vi "Gradient Ascent.vi"(0 "Function":enum16{"Reset", "Ascend"}(ring)=enum."Ascend", 1 "Set Inverse Matrix":T2=[[1.0, 0.0, 0.0], [0.0, 1.0, 0.0], [0.0, 0.0, 1.0]], 5 "Target Data":T1, 7 "Current Data":T1={"Match"={"Position"={"x"=0.0, "y"=0.0}, "Angle"=0.0, "Scale"=0.0, "Score"=0.0, "Bounding Box"=[]}, "Edge Analysis"={"Mean Value"=nan, "Standard Variation"=0.0, "Minimal Value"=0.0, "Maximal Value"=0.0, "Area (calibrated)"=0.0, "Area (pixels)"=0, "%"=0.0}}, 9 "Z":dbl=0.02, 11 "error in (no error)":errorcluster, 12 "Delta Z0":dbl=0.02, 14 "Alpha":dbl=0.01) -> (6 "Position Correction":dbl[](array[numeric]), 10 "Delta Z":dbl, 15 "error out":errorcluster)   [LabVIEW 2014]
uses:
  <vilib>/Analysis/Matrix/Datatypes/RealMatrix.ctl
  <vilib>/Analysis/baseanly.llb/A x Vector.vi
  <vilib>/Analysis/NI_AALBase.lvlib
  <vilib>/Analysis/NI_AALPro.lvlib
  <vilib>/Analysis/Matrix/NI_Matrix.lvlib
panel:
  out "Step Counter":i32
  out "Slope Fit":cluster{"Best Linear Fit":dbl[], sgl[]}[](graph)
  # "LICENSED MATERIALS – PROPERTY OF IBM\nCopyright IBM Corp. 2016, 2016\nALL RIGHTS RESERVED"
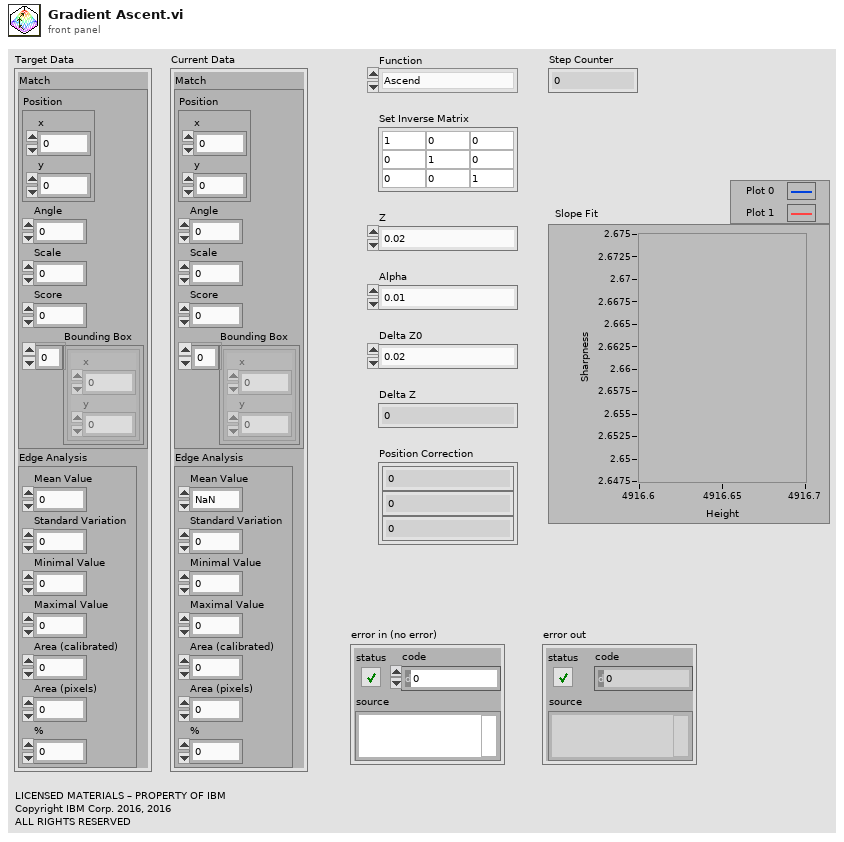
[diagram p1: front panel]
types:
  T1 = cluster{"Match":cluster{"Position":cluster{"x":sgl, "y":sgl}, "Angle":sgl, "Scale":sgl, "Score":sgl, "Bounding Box":cluster{"x":sgl, "y":sgl}[]}, "Edge Analysis":cluster{"Mean Value":sgl, "Standard Variation":sgl, "Minimal Value":sgl, "Maximal Value":sgl, "Area (calibrated)":sgl, "Area (pixels)":i32, "%":sgl}}
  T2 = typedef "NI_Matrix.lvlib/RealMatrix.ctl" = dbl[][]
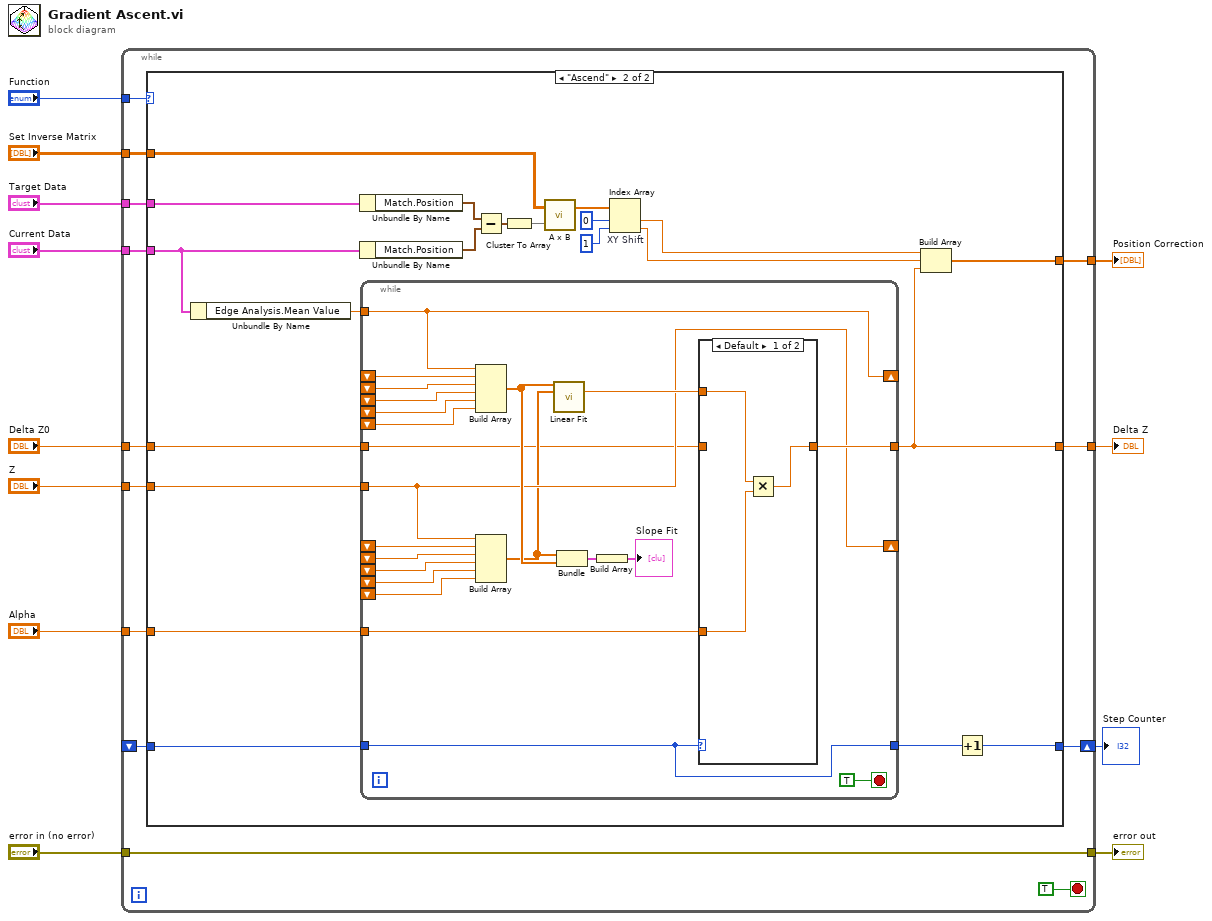
[diagram p0: block diagram]
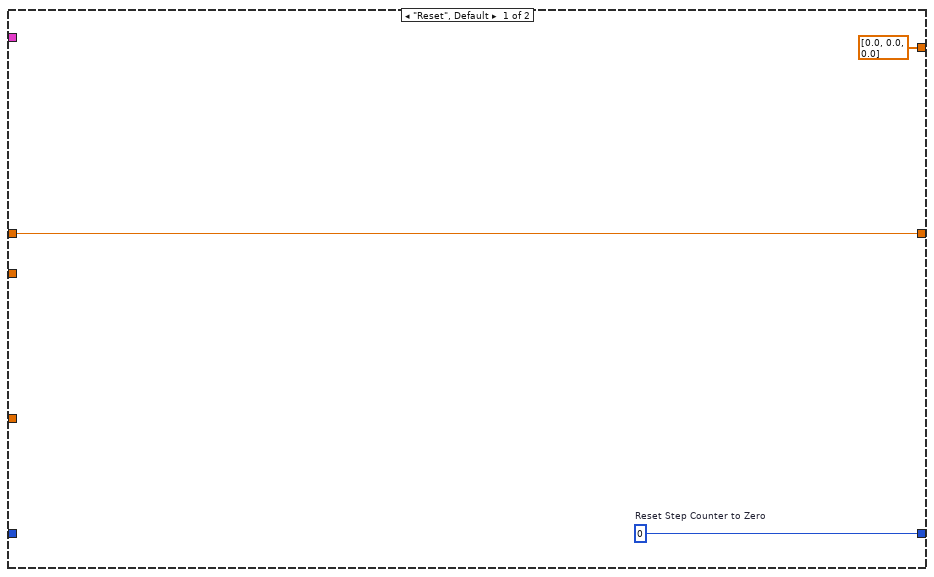
[diagram p2: hidden frame]
diagram:
  n1 = while {
    tunnel: "Set Inverse Matrix" -> [w25]
    tunnel: "Target Data" -> [w24]
    tunnel: "Current Data" -> [w23]
    tunnel: "Alpha" -> [w22]
    tunnel: "Z" -> [w21]
    shift-right: [w16] -> w1
    shift-left: _ -> [w15]
    tunnel: [w19] -> w7
    tunnel: [w18] -> w6
    tunnel: "Function" -> [w17]
    tunnel: "Delta Z0" -> [w14]
    tunnel: [w13] -> w3
    tunnel: "error in (no error)" -> [w13]
    stop <- TRUE stop-if-true
    n2 = case shown="\"Ascend\"" w17 {
      tunnel: w25 -> [_ w49]
      tunnel: w24 -> [_ w48]
      tunnel: w23 -> [_ w47]
      tunnel: w22 -> [_ w46]
      tunnel: w21 -> [_ w35]
      tunnel: [dbl[] [0.0, 0.0, 0.0] w34] -> w19
      tunnel: [w26 w33] -> w18
      tunnel: [w28 w30] -> w16
      tunnel: w15 -> [_ w32]
      tunnel: w14 -> [w26 w29]
      frame "Reset", Default {
        w28 = 0  # Reset Step Counter to Zero
      }
      frame "Ascend" {
        n3 = Unbundle By Name(w47) -> ("Edge Analysis.Mean Value"=w38:sgl)
        n4 = Unbundle By Name(w48) -> ("Match.Position"=w42:cluster{"x":sgl, "y":sgl})
        n5 = Unbundle By Name(w47) -> ("Match.Position"=w40:cluster{"x":sgl, "y":sgl})
        n6 = while {
          shift-right: [w66] -> _
          shift-left: _ -> [w69]
          shift-right: [w62] -> _
          shift-left: _ -> [w61]
          tunnel: w46 -> [w70]
          tunnel: w38 -> [w66]
          tunnel: w32 -> [w51]
          shift-left: _ -> [w68]
          shift-left: _ -> [w60]
          tunnel: [w63] -> w33
          tunnel: w35 -> [w62]
          shift-left: _ -> [w57]
          shift-left: _ -> [w56]
          shift-left: _ -> [w54]
          shift-left: _ -> [w55]
          shift-left: _ -> [w52]
          shift-left: _ -> [w53]
          tunnel: [w51] -> w31
          tunnel: w29 -> [w50]
          stop <- TRUE stop-if-true
          n7 = Build Array(w66, w69, w68, w57, w54, w55) -> (w65:sgl[])
          n8 = Build Array(w62, w61, w60, w56, w52, w53) -> (w59:dbl[])
          n9 = call <vilib>:"Linear Fit.vi"("Y"=w65, "X"=w59) -> ("slope"=w67:dbl)  [unwired: 9 in, 4 out]
          n10 = Bundle(w59, w65) -> (w64:cluster{dbl[], sgl[]})  [unwired: 1 in]
          n11 = Build Array(w64) -> (→"Slope Fit":cluster{dbl[], sgl[]}[])
          n12 = case shown="Default" w51 {
            tunnel: w70 -> [w73 _]
            tunnel: [w74 w75] -> w63
            tunnel: w67 -> [w72 _]
            tunnel: w50 -> [_ w75]
            frame Default {
              n13 = Multiply(x=w72, y=w73) -> (x*y=w74:dbl)
            }
            frame 0..4 {
            }
          }
        }
        n14 = Subtract(x=w42, y=w40) -> (x-y=w44:cluster{"x":sgl, "y":sgl})
        n15 = Cluster To Array(cluster=w44) -> (array=w43:sgl[])
        n16 = call-poly <vilib>:"A x B.vi"("Vector"=w43, "A"=w49) -> ("A x Vector"=w45:dbl[])  [unwired: 1 out]
        n17 = Index Array "XY Shift"(array=w45, index #1=0 ("index"), index #2=1 ("index")) -> (element #1=w37:dbl, element #2=w36:dbl)
        n18 = Build Array(w37, w36, w33) -> (w34:dbl[])
        n19 = Increment(x=w31) -> (x+1=w30:i32)
      }
    }
  }
  "Position Correction" <- w7
  "Delta Z" <- w6
  "error out" <- w3
  "Step Counter" <- w1
